vi "Write Frequency.vi"(8 "error in (no error)":errorcluster, 10 "Frequency":dbl, 11 "Set Frequency Message in":refnum<class "Set Frequency Message.lvclass">) -> (0 "error out":errorcluster, 3 "Set Frequency Message out":refnum<class "Set Frequency Message.lvclass">)   [LabVIEW 2011, in "Set Frequency Message.lvclass"]
uses:
  Set Frequency Message.lvclass
  Set Frequency Message.lvclass/Set Frequency Message.ctl
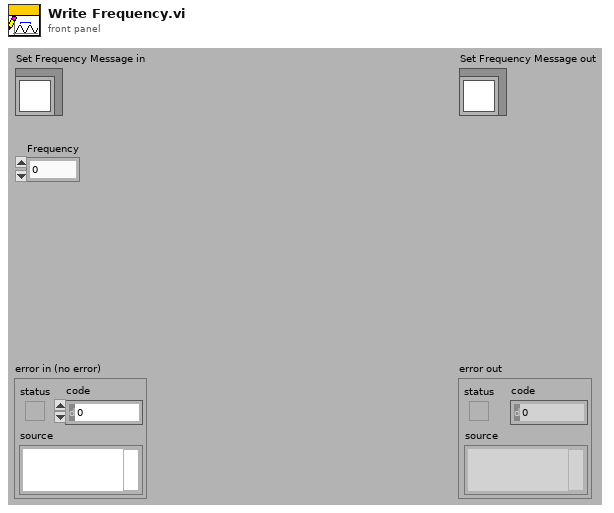
[diagram p1: front panel]
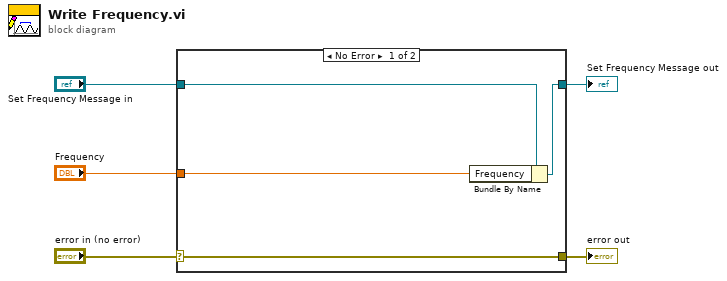
[diagram p0: block diagram]
diagram:
  n1 = case shown="No Error" "error in (no error)" {
    selector: "error in (no error)" -> [w9 w10]
    tunnel: [w9 w10] -> w4
    tunnel: [w7 w11] -> w2
    tunnel: "Set Frequency Message in" -> [w8 w11]
    tunnel: "Frequency" -> [w6 _]
    frame No Error {
      n2 = Bundle By Name(cluster=w8, "Frequency"=w6) -> (w7:refnum<class "Set Frequency Message.lvclass">)
    }
    frame Error {
    }
  }
  "error out" <- w4
  "Set Frequency Message out" <- w2
